vi "Decimation - time to write.vi"(8 "Block descriptors":T1[](array[typedef]), 10 "Iteration":i32, 11 "Decimation":i32) -> (3 "Trigger?":bool)   [LabVIEW 2019, in "RefMem DMA Engine.lvlib"]
uses:
  RefMem DMA Engine.lvlib
  Shared/Block descriptor.ctl
  Shared/RefMem DMA Shared.lvlib
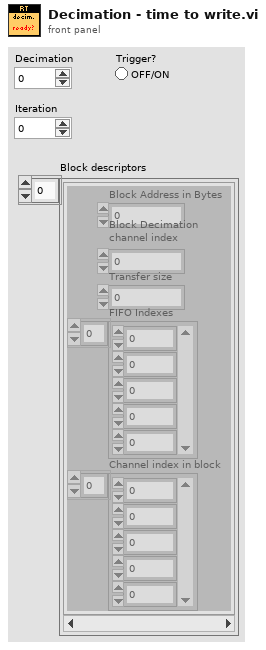
[diagram p1: front panel]
types:
  T1 = typedef "RefMem DMA Shared.lvlib/Block descriptor.ctl" = cluster{"Block Address in Bytes":u32, "Block Decimation \nchannel index":i32, "Transfer size":u32, "FIFO Indexes":i32[], "Channel index in block":i32[]}
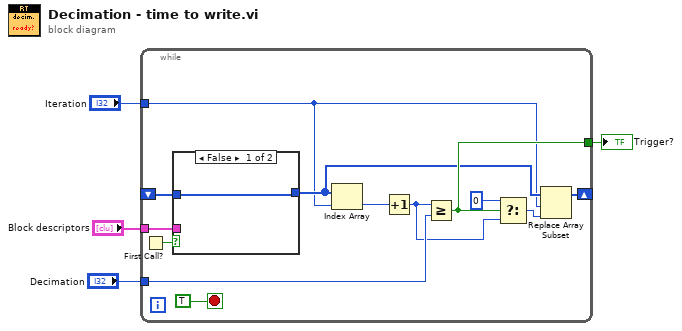
[diagram p0: block diagram]
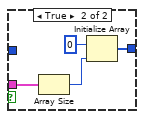
[diagram p2: hidden frame]
diagram:
  n1 = while {
    tunnel: "Block descriptors" -> [w15]
    tunnel: "Iteration" -> [w8]
    tunnel: "Decimation" -> [w13]
    tunnel: [w12] -> w1
    shift-right: [w6] -> _
    shift-left: _ -> [w5]
    stop <- TRUE stop-if-true
    n2 = First Call?() -> (First Call?: T/F=w16:bool)
    n3 = case shown="False" w16 {
      tunnel: w15 -> [_ w22]
      tunnel: [w18 w19] -> w9
      tunnel: w5 -> [w18 _]
      frame False {
      }
      frame True {
        n4 = Array Size(array=w22) -> (size(s)=w21:i32)
        n5 = Initialize Array(0, w21) -> (w19:i32[])
      }
    }
    n6 = Index Array(array=w9, index=w8) -> (element=w14:i32)
    n7 = Increment(x=w14) -> (x+1=w11:i32)
    n8 = Greater Or Equal?(x=w11, y=w13) -> (x >= y?=w12:bool)
    n9 = Select(t=0, s=w12, f=w11) -> (s? t:f=w7:i32)
    n10 = Replace Array Subset(array=w9, new element=w7, index=w8) -> (w6:i32[])
  }
  "Trigger?" <- w1
